vi "Prueba_escritura_config.vi"() -> ()   [LabVIEW 2015]
uses:
  <vilib>/Utility/config.llb/Read Key (Double).vi
  <vilib>/Utility/config.llb/Write Key (Double).vi
  <vilib>/Utility/config.llb/NI_LVConfig.lvlib
panel:
  out "error out 3":errorcluster
  out "value 2":dbl
  out "value":dbl
  out "error out 2":errorcluster
  out "error out":errorcluster
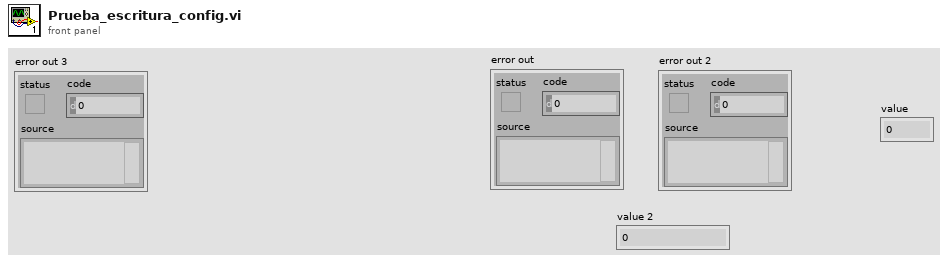
[diagram p1: front panel]
types:
  T1 = typedef "NI_LVConfig.lvlib/Config Data RefNum.ctl" = refnum<k1>
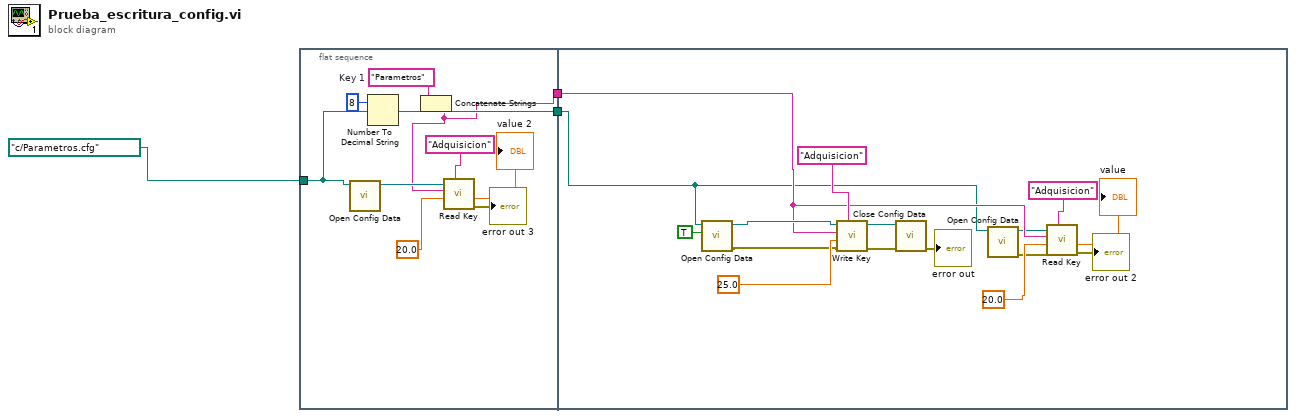
[diagram p0: block diagram]
diagram:
  n1 = flat-sequence {
    tunnel: path "c:/Parametros.cfg" ("configuration file path") -> [w9]
    tunnel: [w9] -> w2
    tunnel: [w4] -> w1
    tunnel: w2 -> [w16]
    tunnel: w1 -> [w20]
    frame #0 {
      w6 = "Parametros"  # Key 1
      n2 = call <vilib>:"Open Config Data.vi"("configuration file path"=w9) -> ("refnum"=w8:T1)  [unwired: 2 in, 8 out]
      n3 = Number To Decimal String(number=8) -> (decimal integer string=w7:string)  [unwired: 1 in]
      n4 = Concatenate Strings(w6, w7) -> (w4:string)
      n5 = call-poly <vilib>:"Read Key.vi"("section"="Adquisicion", "default value"=20.0, "key"=w4, "refnum"=w8) -> ("error out"=→"error out 3":errorcluster, "value"=→"value 2":dbl)  [unwired: 4 in, 2 out]
    }
    frame #1 {
      n6 = call <vilib>:"Open Config Data.vi"("create file if necessary (T)"=TRUE, "configuration file path"=w16) -> ("error out"=w24:errorcluster, "refnum"=w22:T1)  [unwired: 1 in, 7 out]
      n7 = call-poly <vilib>:"Write Key.vi"("section"="Adquisicion", "error in (no error)"=w24, "value"=25.0 ("default value"), "key"=w20, "refnum"=w22) -> ("error out"=w18:errorcluster, "refnum out"=w19:T1)  [unwired: 3 in, 2 out]
      n8 = call <vilib>:"Close Config Data.vi"("error in (no error)"=w18, "refnum"=w19) -> ("error out"=→"error out":errorcluster)  [unwired: 8 in, 1 out]
      n9 = call <vilib>:"Open Config Data.vi"("configuration file path"=w16) -> ("error out"=w15:errorcluster, "refnum"=w14:T1)  [unwired: 2 in, 7 out]
      n10 = call-poly <vilib>:"Read Key.vi"("section"="Adquisicion", "error in (no error)"=w15, "default value"=20.0, "key"=w20, "refnum"=w14) -> ("error out"=→"error out 2":errorcluster, "value"=→"value":dbl)  [unwired: 3 in, 2 out]
    }
  }
